vi "Dashboard Main.vi"() -> ()   [LabVIEW 2017]
uses:
  <vilib>/event_ctls.llb/eventvkey.ctl
  <vilib>/Rock Robotics/WPI/Dashboard/WPI_DashboardLogging Global.vi
  <vilib>/Utility/miscctls.llb/LVRowAndColumnTypeDef.ctl
  Shared/TypeDef/Cluster_Drive_RPM.ctl
  Support/Utility/FP_Size VI to Decoration Simple.vi/TypeDefs_Utility/ENUM RB_Pos_Quadrant Position.ctl
  Support/Utility/FP_Size VI to Decoration Simple.vi/TypeDefs_Utility/Cluster_FP Set.ctl
  RoboRio code/TypeDef/CLUSTER_Drive_Point Specification.ctl
panel:
  in  "Camera Settings Right":T1={"Frame Rate"=30, "Compression"=30, "Size"=1, "DB Camera Config"=FALSE} {"Frame Rate" scale=1.0..30.0; "Compression" scale=100.0..-1.0; "Size" items=["640x480", "320x240", "160x120"]}
  in  "Camera Name Right":string(combo)="No Camera Selection"
  out "Camera Info":cluster{"Mbps LED":bool, "Mbps":dbl, "fps":dbl} {"fps" format="%#.1g"; "Mbps" format="%#.1g"}
  in  "Camera Settings":T1={"Frame Rate"=30, "Compression"=30, "Size"=1, "DB Camera Config"=FALSE} {"Frame Rate" scale=1.0..30.0; "Compression" scale=100.0..-1.0; "Size" items=["640x480", "320x240", "160x120"]}
  in  "TCP":refnum<k5>
  in  "Rec Mode":enum32{"Stop", "Record", "Playback"}(radio)
  out "Robot IP":string
  out "Image Message":string="Timeout in Camera Communications"
  in  "Dashboard Tab":T2(tab)
  in  "Select Auto":string(combo)="Select Autonomous ..."
  out "NT Connection":bool
  out "MotorChart R":cluster{"Numeric":dbl, "Numeric":dbl}(graph)
  out "MotorChart L":cluster{"Numeric":dbl, "Numeric":dbl}(graph)
  out "MotorSliders R":cluster{"MotorSlide1":dbl, "MotorSlide2":dbl} {"MotorSlide2" scale=-1.0..1.0 scale format="%#_2e"; "MotorSlide1" scale=-1.0..1.0 scale format="%#_2e"}
  out "MotorSliders L":cluster{"MotorSlide1":dbl, "MotorSlide2":dbl} {"MotorSlide2" scale=-1.0..1.0 scale format="%#_2e"; "MotorSlide1" scale=-1.0..1.0 scale format="%#_2e"}
  out "Gyro":dbl(knob) scale=0.0..360.0
  out "JS1 Z":dbl(slide) scale=-1.0..1.0 scale format="%#_2e"
  out "JS1 Graph":cluster{"X":dbl, "Y":dbl}[](graph)
  out "JS1 Buttons":T3
  out "JS2 Z":dbl(slide) scale=-1.0..1.0 scale format="%#_2e"
  out "JS2 Graph":cluster{"X":dbl, "Y":dbl}[](graph)
  out "JS2 Buttons":T3
  out "Mode":T4(ring)=enum."Auto Disabled"
  out "Camera Image Right":T5(plugin-control)
  in  "DB/String 9":string
  in  "DB/String 8":string
  in  "DB/String 7":string
  in  "DB/String 6":string
  in  "DB/String 5":string
  in  "DB/String 4":string
  in  "DB/String 3":string
  in  "DB/String 2":string
  in  "DB/String 1":string
  in  "DB/String 0":string
  in  "DB/Slider 0":dbl(slide) scale=0.0..5.0
  in  "DB/Slider 1":dbl(slide) scale=0.0..5.0
  in  "DB/Slider 2":dbl(slide) scale=0.0..5.0
  in  "DB/Slider 3":dbl(slide) scale=0.0..5.0
  out "DB/LED 3":bool
  out "DB/LED 2":bool
  out "DB/LED 1":bool
  out "DB/LED 0":bool
  in  "DB/Button 3":bool
  in  "DB/Button 2":bool
  in  "DB/Button 1":bool
  in  "DB/Button 0":bool caption="New Name"
  out "Low Gear":bool
  out "High Gear":bool
  out "Drive Mode":enum16{"Motion Profile", "VBus", "Stop"}(ring)
  out "Profile Enabled":bool
  out "Turbo Enabled":bool
  out "VBus X":dbl
  out "VBus Y":dbl
  out "Right Encoder":dbl
  out "Left Encoder":dbl
  out "Comp. Running":bool
  out "Comp. Enabled":bool
  in  "Reset Max RPM":bool
  out "Right Max":dbl
  out "Left Max":dbl
  out "Right":dbl
  out "Left":dbl
  out "Left Front":dbl
  out "Right Back":dbl
  out "Right Front":dbl
  out "Left Back":dbl
  out "Battery Meter":dbl(knob) scale=0.0..15.0
  out "Solenoid":bool[](array[boolean])
  out "Batt V":bool
  out "Temp":bool
  out "HW":bool
  out "Comp.":bool
  out "Voltage(V)":dbl
  out "Power (W)":dbl
  out "Energy (J)":dbl
  out "Input (V)":dbl
  out "Solenoid (V)":dbl
  out "Current (A)":dbl
  out "5V Usr. Rail Brn.":bool
  out "Input Brn.":bool
  out "6V":bool
  out "3.3V":bool
  out "5V":bool
  out "?":T6(graph)
  out "?":T6(graph)
  out "PDP Currents":string[][](table)
  in  "Profule Array":T7[](array[typedef])
  in  "Send Profile to RIO":bool
  out "Import Successful":bool
  in  "Prifile File Path on PC":path
  in  "Import File":bool
  in  "Test Slider":dbl(slide) scale=0.0..100.0 scale format="%#_3g"
  in  "On/Off":bool caption="Solenoid"
  in  "Test Name":u16(ring) items=["Select the test to run..."]
  in  "Test Tree":string(tree)
  in  "Motor":cluster{"Value":dbl, "Enable":bool} {"Value" scale=-1.0..1.0 scale format="%#_3g"}
  out "Progress":T8 {"Test Progress" scale=0.0..100.0}
  in  "Rev/Fwd":cluster{"Forward":bool, "Reverse":bool}
  in  "Test Ring":u16(ring) items=["Monochrome", "Color"]
  out "Cmd Status":string
  in  "Execute Command":bool
  in  "Command Params":string[][](table)
  in  "Command Selection":i32(listbox)
  in  "CheckList":i32(listbox)
  out "Tree":string(tree)
  out "Camera Image":T5(plugin-control)
  in  "Camera Name":string(combo)="No Camera Selection"
  # "HW"
  # "HW"
  # "Joysticks"
  # "Drive Motors"
  # "Front"
  # "Right"
  # "Left"
  # "Back"
  # "SRX Currents"
  # "Drive RPMs"
  # "Drive"
  # "Faults"
  # "PDP"
  # "PCM"
  # "RIO Faults"
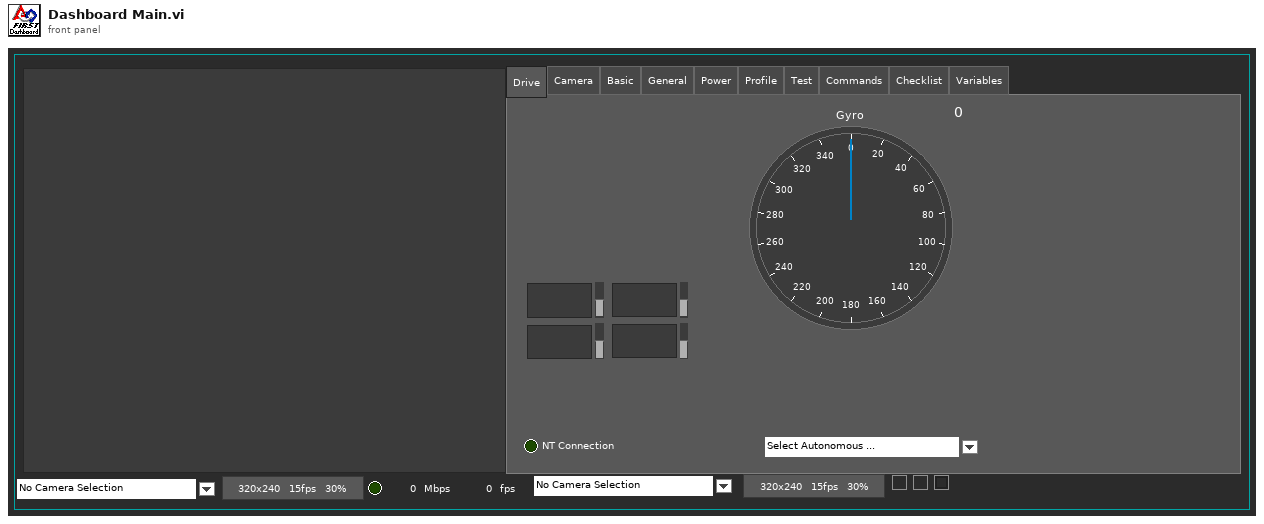
[diagram p1: front panel]
types:
  T1 = cluster{"Frame Rate":i32, "Compression":i32, "Size":u16, "DB Camera Config":bool}
  T2 = enum32{"Drive", "Camera", "Basic", "General", "Power", "Profile", "Test", "Commands", "Checklist", "Variables"}
  T3 = cluster{bool, bool, bool, bool, bool, bool, bool, bool, bool, bool, bool, bool}
  T4 = enum8{"Tele-Op Disabled", "Tele-Op Enabled", "Auto Disabled", "Auto Enabled", "Test Disabled", "Test Enabled", "Disconnected", "No Code", "E-Stop"}
  T5 = typedef "IMAQ Image.ctl" = refnum<image>
  T6 = cluster{"Vol.  (V)":dbl, "Vol.  (V)":dbl, "Vol.  (V)":dbl}
  T7 = typedef "CLUSTER_Drive_Point Specification.ctl" = cluster{"Position":dbl, "Velocity":dbl, "Duration ms":u8}
  T8 = cluster{"Test Progress":u8, "Test Progress Text":string}
  T9 = cluster{"Operation":enum16{"Update", "Clear"}, "Color Box":u32}[]
  T10 = typedef "Image Type" = u32
  T11 = cluster{"IDs":cluster{"RPC field ID":u16, "Unique ID":u16}, "String":string}
  T12 = enum32{"Drive", "Basic", "Custom", "Test", "Checklist", "Variables"}
  T13 = cluster{"Camera Image":refnum<vi>, "Dashboard Tab":refnum<vi>, "Rec Mode":refnum<vi>, "Test Slider":refnum<vi>, "On/Off ":refnum<vi>, "Test Ring":refnum<vi>, "Rev/Fwd":refnum<vi>, "Test Name":refnum<vi>, "Motor":refnum<vi>, "Progress":refnum<vi>, "CheckList":refnum<vi>, "Tree":refnum<vi>, "Test Tree":refnum<vi>, "Command Params":refnum<vi>, "Command Selection":refnum<vi>, "Execute Command":refnum<vi>, "Cmd Status":refnum<vi>, "Camera Settings":refnum<vi>, "Camera Name":refnum<vi>, "Camera Info":refnum<vi>, "Camera Settings Right":refnum<vi>, "Camera Name Right":refnum<vi>, "Camera Image Right":refnum<vi>}
  T14 = typedef "Cluster_FP Set.ctl" = cluster{"Menu Bar":bool, "Position":T15, "Decoration index":i32, "border(px)":i32, "Monitor #":i32}
  T15 = typedef "ENUM RB_Pos_Quadrant Position.ctl" = enum32{"LFT-TOP", "MID-TOP", "RGT-TOP", "LFT-CTR", "MID-CTR", "RGT-CTR", "LFT-BOT", "MID-BOT", "RGT-BOT"}
  T16 = typedef "Cluster_Drive_RPM.ctl" = cluster{"Left Side":dbl, "Right Side":dbl}
  T17 = typedef "LVRowAndColumnTypeDef.ctl" = cluster{"Row":i32, "Column":i32}
  T18 = cluster{"Error Strings":string, "Disable Counts":cluster{u16, u16}, "Rail Faults":cluster{u16, u16, u16}, "Robot IP":string, "DB Mode":u8, "Event Info":cluster{"Name":string, "Type":u8, "Number":u16, "Replay":u8}}
  T19 = cluster{"Storage":cluster{"Disk Free":u64, "RAM Block":u32, "RAM free":u32}, "CPU Utilization":cluster{"CPU % ISR":sgl, "CPU % Time Crit":sgl, "CPU % Timed Str":sgl, "CPU % High":sgl, "CPU % Above":sgl, "CPU % Normal":sgl, "CPU % Low":sgl}, "CAN":cluster{"% Bus Utilization":sgl, "Bus Off Cnt":u32, "TX_FIFO Full Cnt":u32, "Receive Error Cnt":u8, "Transmit Error Cnt":u8}, "HID":cluster{"HID Outputs":u32, "Rumble Low":u16, "Rumble High":u16}[]}
  T20 = cluster{"Status bits":cluster{"Test Mode":bool, "Autonomous":bool, "Enabled":bool, "Code Start":bool, "Brownout":bool, "Reserved 2":bool, "Reserved 3":bool, "E-Stop":bool}, "Code Trace":cluster{"Disabled":bool, "TeleOp":bool, "Auto":bool, "Test":bool}, "Controller Type":enum16{"unknown", "cRIO", "roboRio"}, "Code?":enum16{"unknown", "noCode", "code"}, "Battery V":dbl}
  T21 = cluster{"Control Bits":cluster{"TestMode":bool, "Autonomous":bool, "Enabled":bool, "FMS Present":bool, bool, bool, bool, "E-Stop":bool}, "Team Station ":u8, "Countdown":sgl, "Joystick Values":cluster{"Axes":dbl[], "Buttons":bool[], "POVs":i16[]}[]}
  T22 = cluster{"Axes":dbl[], "Buttons":bool[], "POVs":i16[]}[]
  T23 = typedef "CLUSTER_PDP_Status.ctl" = cluster{"PDP Faults":T24, "All Currents (A)":dbl[], "Energy (J)":dbl, "Power (W)":dbl, "Voltage (V)":dbl}
  T24 = typedef "CLUSTER_PDP_Faults.ctl" = cluster{"Current Faults":bool[], "Batt V Fault":bool, "Temp Fault":bool, "HW Fault":bool}
  T25 = typedef "CLUSTER_PCM_Status.ctl" = cluster{"Current (A)":dbl, "All Solenoid Faults":bool[], "Input Voltage":dbl, "Solenoid Voltage":dbl, "Comp. Fault":bool}
  T26 = typedef "CLUSTER_RoboRio_Status.ctl" = cluster{"RoboRio Faults":T27, "RIO inpt vol (V)":dbl, "RIO inpt cur (A)":dbl, "RoboRio Rails":T28}
  T27 = typedef "CLUSTER_RoboRio_Faults.ctl" = cluster{"Inpt. V. Brn. Out":bool, "3.3V Usr Rail Shrt.":bool, "5 V Usr Rail Shrt.":bool, "6 V Usr. Rail Shrt.":bool, "5V Usr. Rail Brn. Out":bool}
  T28 = typedef "CLUSTER_RoboRio_Rails.ctl" = cluster{"3.3 Volt":T29, "5 Volt":T29, "6 Volt":T29}
  T29 = typedef "CLUSTER_RoboRio_SingleRail.ctl" = cluster{"Vol.  (V)":dbl, "Cur. (A)":dbl}
  T30 = cluster{"Axes":dbl[], "Buttons":bool[], "POVs":i16[]}
  T31 = cluster{"Buttons[0]":bool, "Buttons[1]":bool, "Buttons[2]":bool, "Buttons[3]":bool, "Buttons[4]":bool, "Buttons[5]":bool, "Buttons[6]":bool, "Buttons[7]":bool, "Buttons[8]":bool, "Buttons[9]":bool, "Buttons[10]":bool, "Buttons[11]":bool}
  T32 = cluster{"Cur. (A)":dbl, "Cur. (A)":dbl, "Cur. (A)":dbl}
  T33 = typedef "Cluster_SRX_Amperage.ctl" = cluster{"Left Back":dbl, "Right Front":dbl, "Right Back":dbl, "Left Front":dbl}
  T34 = typedef "Cluster_Compressor.ctl" = cluster{"Compressor Running":bool, "Compressor Enabled":bool}
  T35 = typedef "Cluster_Encoder_Count.ctl" = cluster{"Left Side Encoder":dbl, "Right Side Encoder":dbl}
  T36 = typedef "CLUSTER_CMD_WC_Drive.ctl" = cluster{"Drive_Mode":T37, "VBus":T38, "Profile":T40}
  T37 = typedef "ENUM_WC_Drive_DriveMode.ctl" = enum16{"Motion Profile", "VBus", "Stop"}
  T38 = typedef "CLUSTER_Drive_ACT Loop_VBus Data.ctl" = cluster{"Drive":T39, "Turbo":bool}
  T39 = typedef "CLUSTER_X and Y.ctl" = cluster{"Steer":dbl, "Throtle":dbl}
  T40 = typedef "CLUSTER_Drive_ACT Loop_Profile Data.ctl" = cluster{"Start":bool}
  T41 = cluster{"Command Params":string[][], "Test Mode Array":cluster{"Operation":enum16{"Update", "Clear"}, "Color Box":u32}[]}
  T42 = typedef "eventvkey.ctl" = enum16{"ASCII", "Enter", "Return", "Shift", "Ctrl", "Alt", "Cmd", "Opt", "Caps", "NumLock", "Clear", "Break", "Up", "Down", "Left", "Right", "Insert", "Delete", "Home", "End", "PageUp", "PageDown", "Escape", "Help", "Pause", "ScrollLock", "F1", "F2", "F3", "F4", "F5", "F6", "F7", "F8", "F9", "F10", "F11", "F12", "F13", "F14", "F15", "F16", "F17", "F18", "F19", "F20", "F21", "F22", "F23", "F24", "Play", "VolumeUp", "VolumeDown", "Mute", "Two Byte Char"}
  T43 = cluster{"Image Size":bool, "Image Type":bool, "Pixel Value":bool, "ROI Information":bool, "Zoom Factor":bool}
  T44 = cluster{"Operation":enum16{"Update", "Clear"}, "Color Box":u32}
  T45 = cluster{"Shift":bool, "Ctrl":bool, "Alt":bool, "Cmd":bool, "Opt":bool}
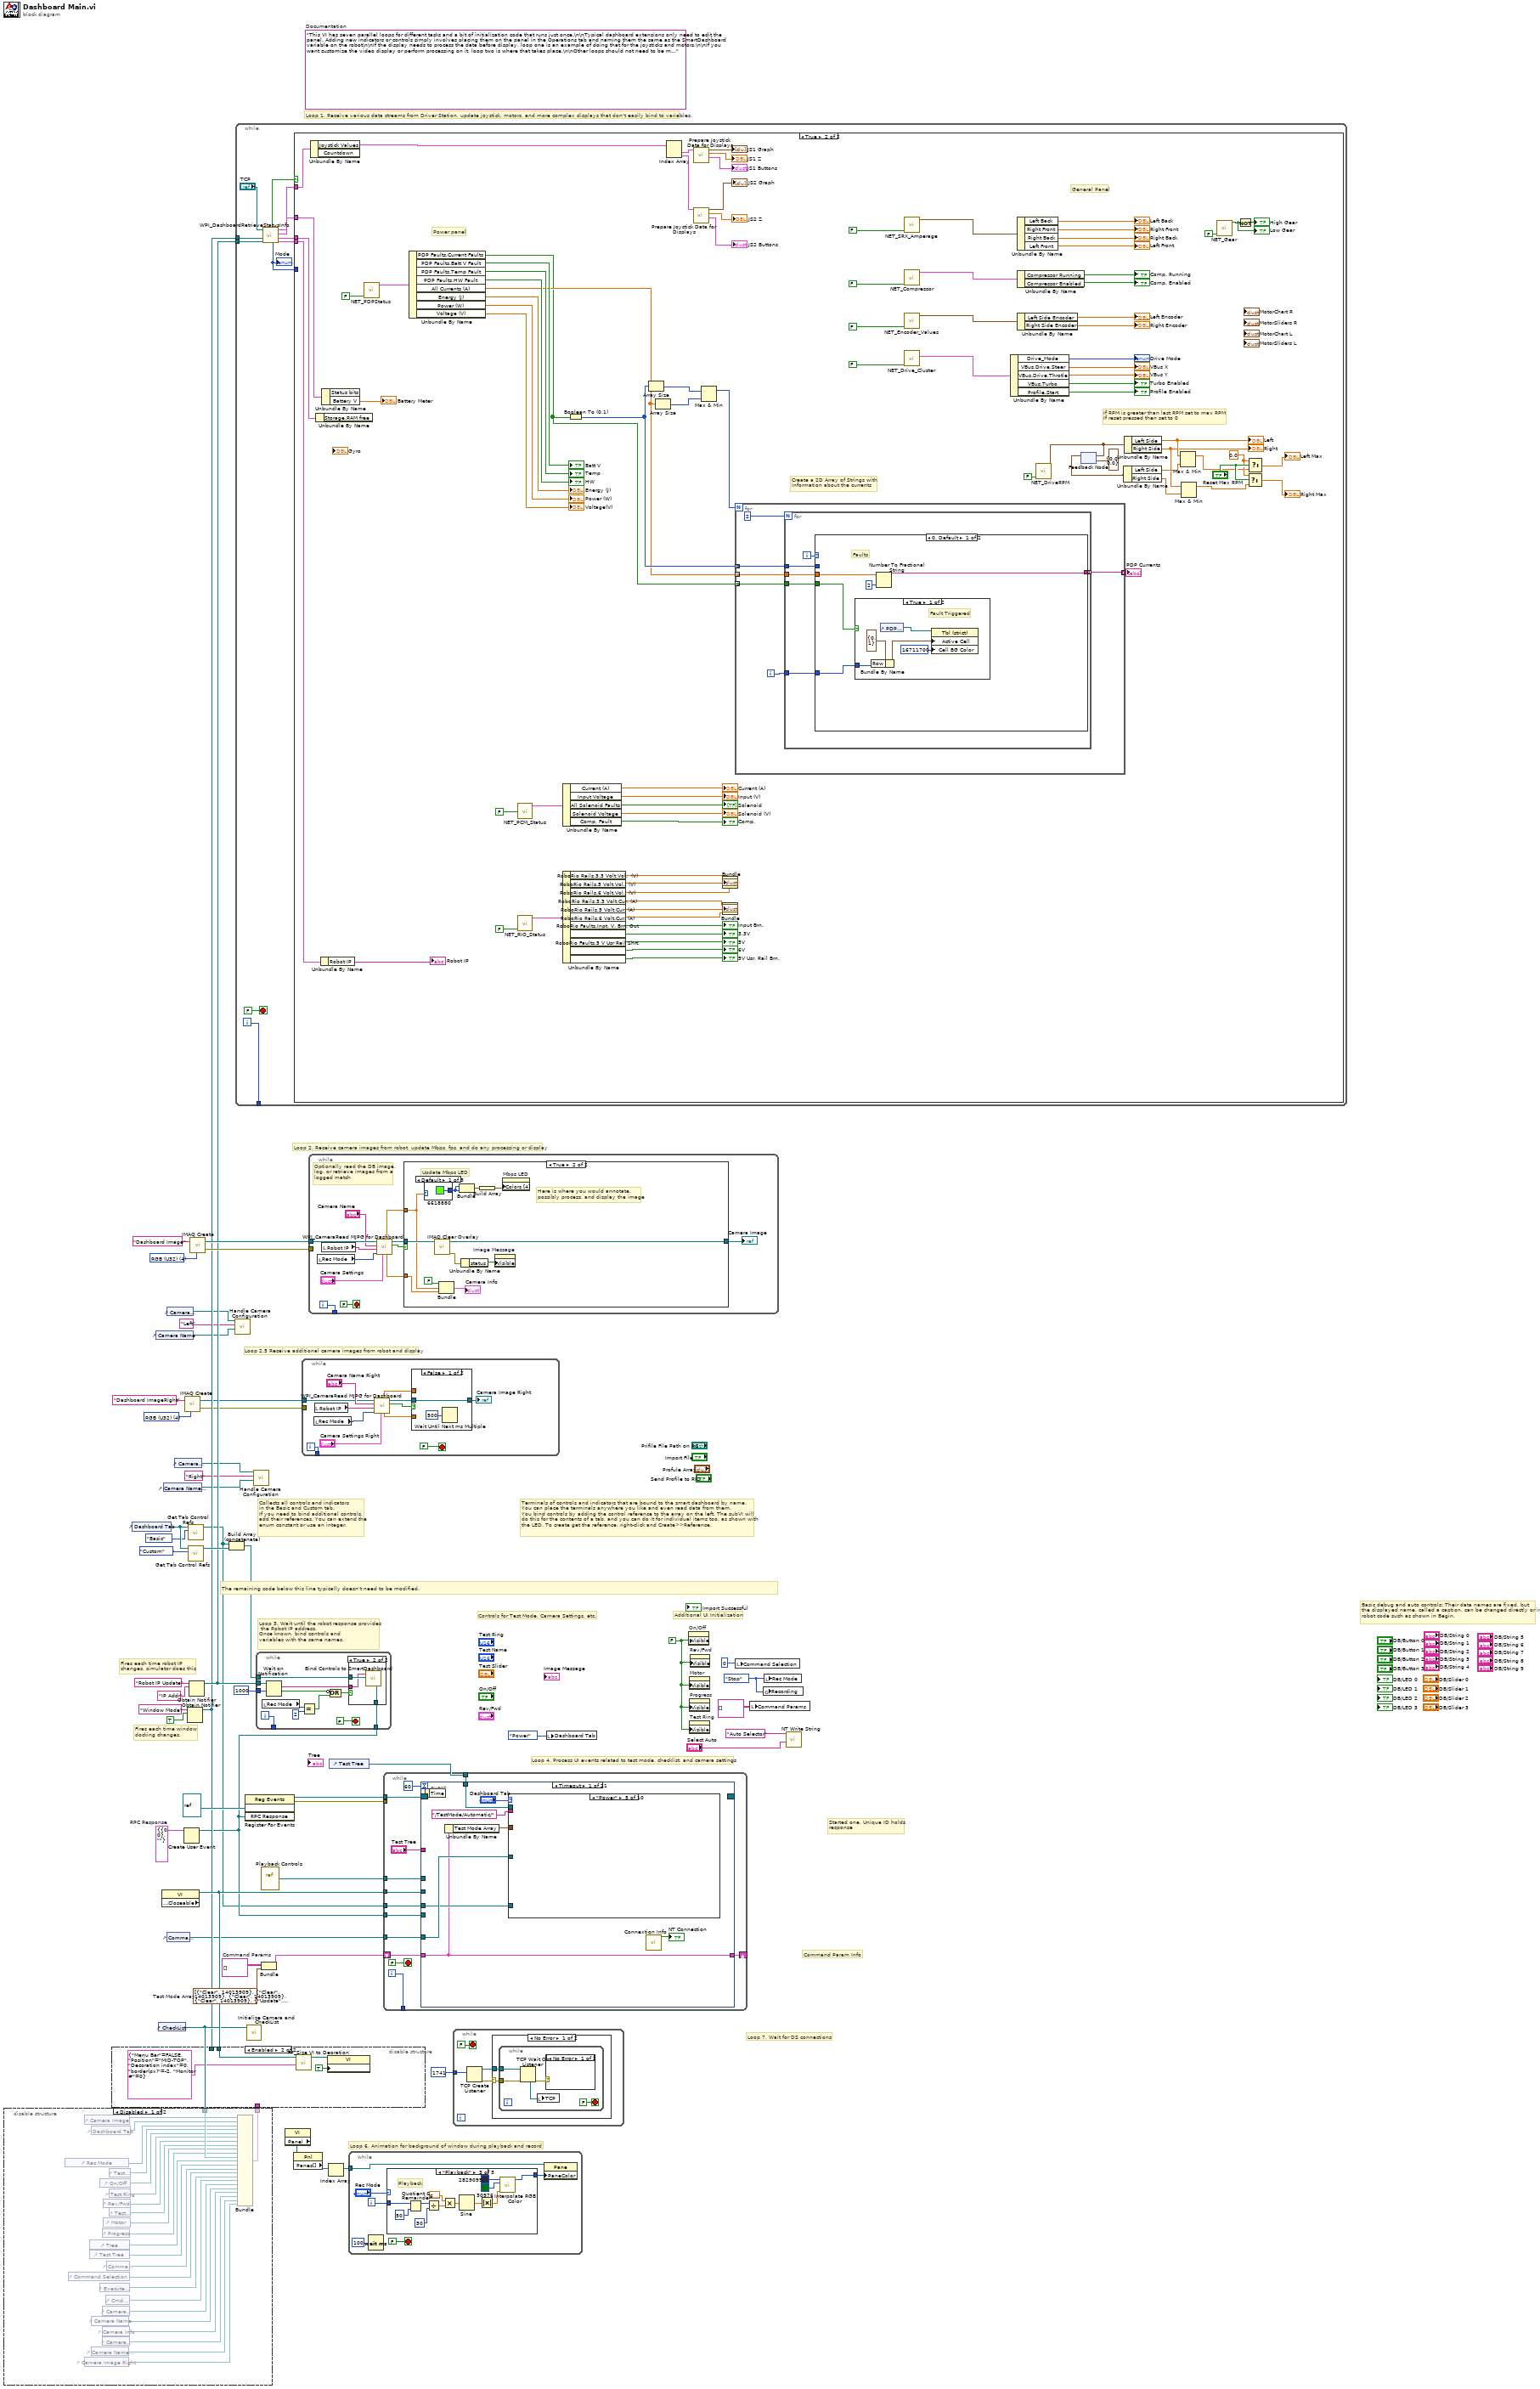
[diagram p0: block diagram]
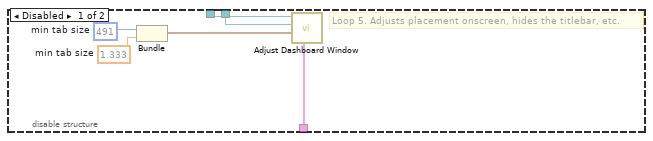
[diagram p2: hidden frame]
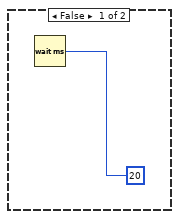
[diagram p5: hidden frame]
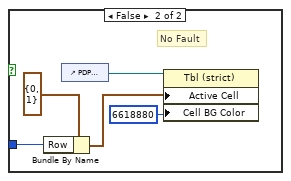
[diagram p6: hidden frame]
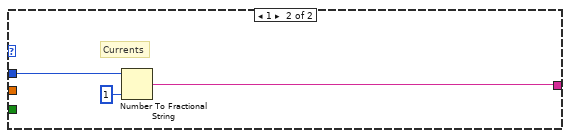
[diagram p7: hidden frame]
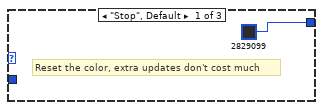
[diagram p8: hidden frame]
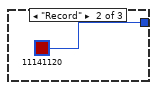
[diagram p9: hidden frame]
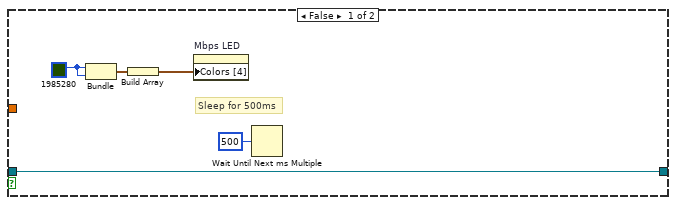
[diagram p11: hidden frame]
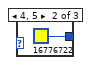
[diagram p12: hidden frame]
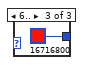
[diagram p13: hidden frame]
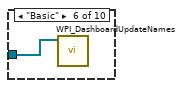
[diagram p18: hidden frame]
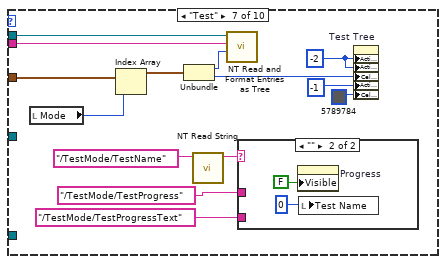
[diagram p19: hidden frame]
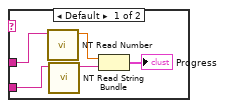
[diagram p20: hidden frame]
diagram:
  w2 = T9 [{"Operation"=enum."Clear", "Color Box"=14013909}, {"Operation"=enum."Clear", "Color Box"=14013909}, {"Operation"=enum."Clear", "Color Box"=14013909}, {"Operation"=enum."Clear", "Color Box"=14013909}, {"Operation"=enum."Update", "Color Box"=14013909}, {"Operation"=enum."Update", "Color Box"=16777215}, {"Operation"=enum."Clear", "Color Box"=14013909}, {"Operation"=enum."Clear", "Color Box"=14013909}, {"Operation"=enum."Clear", "Color Box"=14013909}]  # Test Mode Array
  w4 = string[][] []  # Command Params
  w11 = T10 4 items=["Grayscale (U8)", "Grayscale (I16)", "Grayscale (SGL)", "Complex (CSG)", "RGB (U32)", "HSL (U32)", "RGB (U64)"] ("Image Type")
  w22 = T11 {"IDs"={"RPC field ID"=0, "Unique ID"=0}, "String"=""}  # RPC Response
  w35 = enum32{"Stop", "Record", "Playback"}."Stop" ("Rec Mode")
  w26 = FALSE ("Visible")
  (unwired) "This VI has seven parallel loops for different tasks and a bit of initialization code that runs just once.\n\nTypical dashboard extensions only need to edit the panel. Adding new indicators or controls simply involves placing them on the panel in the Operations tab and naming them the same as the SmartDashboard variable on the robot\n\nIf the display needs to process the data before display, loop one is an example of doing that for the joysticks and motors.\n\nIf you want customize the video display or perform processing on it, loop two is where that takes place.\n\nOther loops should not need to be modified. They are pretty standard, and document the task they perform."  # Documentation
  w52 = T10 4 items=["Grayscale (U8)", "Grayscale (I16)", "Grayscale (SGL)", "Complex (CSG)", "RGB (U32)", "HSL (U32)", "RGB (U64)"] ("Image Type")
  # "Loop 2.5 Receive additional camera images from robot and display"
  # "Command Param Info"
  # "Started one, Unique ID holds\nresponse"
  # "Loop 7. Wait for DS connections"
  # "Basic debug and auto controls: Their data names are fixed, but\nthe displayed name, called a caption, can be changed directly or in\nrobot code such as shown in Begin."
  # "Controls for Test Mode, Camera Settings, etc."
  # "Additional UI Initialization"
  # "Loop 6. Animation for background of window during playback and record"
  # "Fires each time robot IP\nchanges, simulator does this"
  # "Fires each time window\ndocking changes."
  # "Collects all controls and indicators\nin the Basic and Custom tab.\nIf you need to bind additional controls,\nadd their references. You can extend the\nenum constant or use an integer."
  # "The remaining code below this line typically doesn't need to be modified."
  # "Loop 4. Process UI events related to test mode, checklist, and camera settings"
  # "Terminals of controls and indicators that are bound to the smart dashboard by name.\nYou can place the terminals anywhere you like and even read data from them.\nYou bind controls by adding the control reference to the array on the left. The subVI will\ndo this for the contents of a tab, and you can do it for individual items too, as shown with\nthe LED. To create get the reference, right-click and Create>>Reference."
  # "Loop 3. Wait until the robot response provides\n the Robot IP address.\nOnce known, bind controls and\nvariables with the same names."
  # "Loop 1. Receive various data streams from Driver Station, update joystick, motors, and more complex displays that don't easily bind to variables."
  # "Loop 2. Receive camera images from robot, update Mbps, fps, and do any processing or display"
  n1 = control-ref of="Dashboard Tab"() -> (w33:refnum<vi>)
  n2 = control-ref of="Camera Name"() -> (w16:refnum<vi>)
  n3 = control-ref of="CheckList"() -> (w27:refnum<vi>)
  n4 = disable-structure shown="Disabled" {
    disable-tunnel: [w74 _] -> w28
    disable-tunnel: w27 -> [w73 _]
    frame Disabled {
      n5 = control-ref of="Rec Mode"() -> (w68:refnum<vi>)
      n6 = control-ref of="Command Selection"() -> (w60:refnum<vi>)
      n7 = control-ref of="Camera Image Right"() -> (w53:refnum<vi>)
      n8 = control-ref of="Camera Image"() -> (w76:refnum<vi>)
      n9 = control-ref of="Tree"() -> (w72:refnum<vi>)
      n10 = control-ref of="Test Tree"() -> (w71:refnum<vi>)
      n11 = control-ref of="Dashboard Tab"() -> (w75:refnum<vi>)
      n12 = control-ref of="Camera Name"() -> (w57:refnum<vi>)
      n13 = control-ref of="Camera Name Right"() -> (w54:refnum<vi>)
      n14 = control-ref of="Execute Command"() -> (w61:refnum<vi>)
      n15 = control-ref of="On/Off"() -> (w66:refnum<vi>)
      n16 = control-ref of="Progress"() -> (w63:refnum<vi>)
      n17 = control-ref of="Camera Settings"() -> (w58:refnum<vi>)
      n18 = control-ref of="Camera Info"() -> (w56:refnum<vi>)
      n19 = control-ref of="Camera Settings Right"() -> (w55:refnum<vi>)
      n20 = control-ref of="Rev/Fwd"() -> (w64:refnum<vi>)
      n21 = control-ref of="Motor"() -> (w69:refnum<vi>)
      n22 = control-ref of="Cmd Status"() -> (w59:refnum<vi>)
      n23 = control-ref of="Command Params"() -> (w62:refnum<vi>)
      n24 = control-ref of="Test Slider"() -> (w67:refnum<vi>)
      n25 = control-ref of="Test Ring"() -> (w65:refnum<vi>)
      n26 = control-ref of="Test Name"() -> (w70:refnum<vi>)
      n27 = Bundle("Camera Image"=w76, "Dashboard Tab"=w75, "Rec Mode"=w68, "Test Slider"=w67, "On/Off"=w66, "Test Ring"=w65, "Rev/Fwd"=w64, "Test Name"=w70, "Motor"=w69, "Progress"=w63, "CheckList"=w73, "Tree"=w72, "Test Tree"=w71, "Command Params"=w62, "Command Selection"=w60, "Execute Command"=w61, "Cmd Status"=w59, "Camera Settings"=w58, "Camera Name"=w57, "Camera Info"=w56, "Camera Settings Right"=w55, "Camera Name Right"=w54, "Camera Image Right"=w53) -> (w74:T13)  [unwired: 1 in]
    }
    frame Enabled {
    }
  }
  n28 = property class="VI" props=["Front Panel.Closeable"]() -> (reference out=w34:refnum<vi>)  [unwired: 2 in, 2 out]
  n29 = control-ref of="Camera Name Right"() -> (w7:refnum<vi>)
  n30 = control-ref of="Camera Settings"() -> (w17:refnum<vi>)
  n31 = control-ref of="Command Params"() -> (w18:refnum<vi>)
  n32 = control-ref of="Camera Settings Right"() -> (w8:refnum<vi>)
  n33 = Create User Event(user event datatype=w22) -> (user event=w19:refnum<user-event>)  [unwired: 1 in, 1 out]
  n34 = call "IMAQ Create"("Image Name"="Dashboard ImageRight", "Image Type"=w11) -> ("New Image"=w10:T5, "error out"=w9:errorcluster)  [unwired: 2 in, 1 out]
  n35 = Obtain Notifier(name (unnamed)="Window Mode", notification data type=TRUE) -> (notifier out=w24:refnum<notifier>)  [unwired: 2 in, 2 out]
  n36 = disable-structure shown="Enabled" {
    disable-tunnel: w34 -> [w82 w86]
    disable-tunnel: w28 -> [w78 _]
    disable-tunnel: w24 -> [w77 _]
    frame Disabled {
      w81 = 491  # min tab size
      w80 = 1.333  # min tab size
      # "Loop 5. Adjusts placement onscreen, hides the titlebar, etc."
      n37 = Bundle("min tab size"=w81, "min tab size"=w80) -> (w79:cluster{"min tab size":i32, "min tab size":dbl})  [unwired: 1 in]
      n38 = call "Adjust Dashboard Window.vi"("Sizing Refnums"=w78, "Size Constraints"=w79, "VI"=w82, "WIn Mode"=w77) -> ()  [unwired: 8 in]
    }
    frame Enabled {
      n39 = call "FP_Size VI to Deoration.vi"("FPSet"=T14 {"Menu Bar"=FALSE, "Position"=enum."MID-TOP", "Decoration index"=0, "border(px)"=-2, "Monitor #"=0}, "VI Ref"=w86) -> ("VI Ref Out"=w84:refnum<vi>)  [unwired: 8 in, 1 out]
      n40 = property class="VI"(reference=w84, "Front Panel.IsFrontmost"=TRUE ("Front Panel Window:Is Frontmost")) -> ()  [unwired: 1 in, 2 out]
    }
  }
  n41 = call <vilib>:"Get Tab Control Refs.vi"("Page Index"=T12."Basic" ("Dashboard Tab"), "TabControl in"=w33) -> ("ControlsOnPage"=w15:refnum<vi>[])  [unwired: 9 in]
  n42 = call <vilib>:"Get Tab Control Refs.vi"("Page Index"=T12."Custom" ("Dashboard Tab"), "TabControl in"=w33) -> ("ControlsOnPage"=w32:refnum<vi>[])  [unwired: 9 in]
  n43 = Obtain Notifier(name (unnamed)="Robot IP Update", notification data type="IP Addr" ("name (unnamed)")) -> (notifier out=w25:refnum<notifier>)  [unwired: 2 in, 2 out]
  n44 = call "IMAQ Create"("Image Name"="Dashboard Image", "Image Type"=w52) -> ("New Image"=w50:T5, "error out"=w49:errorcluster)  [unwired: 2 in, 1 out]
  n45 = Build Array (concatenate)(w15, w32) -> (w31:refnum<vi>[])
  n46 = call "Handle Camera Configuration.vi"("CameraNameRef"=w16, "Camera File Name"="Left", "ClusterRef"=w17) -> ()  [unwired: 9 in]
  n47 = while {
    tunnel: [w96] -> _
    tunnel: w25 -> [w90]
    tunnel: w24 -> [w87]
    i -> [w96]
    stop <- FALSE stop-if-true
    n48 = call <vilib>:"WPI_DashboardRetrieveStatusInfo.vi"("Binding Refnum"=w90, "Window Mode Notifier"=w87, "TCP Cnx"="TCP") -> ("Power and Errors"=w91:T18, "Robot Metrics"=w94:T19, "Status Info"=w95:T20, "Control Info"=w92:T21, "Robot Mode"=w89:T4, "Process?"=w93:bool)  [unwired: 3 in]
    "Mode" <- w89
    n49 = case shown="True" w93 {
      tunnel: w95 -> [_ w188]
      tunnel: w94 -> [_ w187]
      tunnel: w92 -> [_ w186]
      tunnel: w91 -> [_ w185]
      tunnel: w89 -> [_ _]
      frame False {
        n50 = Wait (ms)(milliseconds to wait=u32 20) -> ()  [unwired: 1 out]
      }
      frame True {
        w108 = 0.0 ("t")
        # "Power panel"
        # "Create a 2D Array of Strings with \ninformation about the currents"
        # "General Panel"
        # "If RPM is greater than last RPM set to max RPM\nIf reset pressed then set to 0"
        n51 = Unbundle By Name(w186) -> ("Joystick Values"=w184:T22)  [unwired: 1 out]
        n52 = Unbundle By Name(w187) -> ()  [unwired: 1 out]
        n53 = Unbundle By Name(w185) -> ("Robot IP"=→"Robot IP":string)
        n54 = Unbundle By Name(w188) -> ("Battery V"=→"Battery Meter":dbl)  [unwired: 1 out]
        n55 = call "NET_PDPStatus.vi"("Read(F) Write(T)"=FALSE) -> ("PDP_Status_Out"=w146:T23)  [unwired: 10 in]
        n56 = Unbundle By Name(w146) -> ("PDP Faults.Current Faults"=w115:bool[], "PDP Faults.Batt V Fault"=→"Batt V":bool, "PDP Faults.Temp Fault"=→"Temp":bool, "PDP Faults.HW Fault"=→"HW":bool, "All Currents (A)"=w137:dbl[], "Energy (J)"=→"Energy (J)":dbl, "Power (W)"=→"Power (W)":dbl, "Voltage (V)"=→"Voltage(V)":dbl)
        n57 = call "NET_PCM_Status.vi"("Read(F) Write(T)"=FALSE) -> ("PCM_Status_Out"=w152:T25)  [unwired: 10 in]
        n58 = call "NET_RIO_Status.vi"("Read(F) Write(T)"=FALSE) -> ("RoboRio Status Out"=w162:T26)  [unwired: 10 in]
        n59 = Unbundle By Name(w152) -> ("Current (A)"=→"Current (A)":dbl, "Input Voltage"=→"Input (V)":dbl, "All Solenoid Faults"=→"Solenoid":bool[], "Solenoid Voltage"=→"Solenoid (V)":dbl, "Comp. Fault"=→"Comp.":bool)
        n60 = Unbundle By Name(w162) -> ("RoboRio Rails.3.3 Volt.Vol.  (V)"=w166:dbl, "RoboRio Rails.5 Volt.Vol.  (V)"=w165:dbl, "RoboRio Rails.6 Volt.Vol.  (V)"=w164:dbl, "RoboRio Rails.3.3 Volt.Cur. (A)"=w160:dbl, "RoboRio Rails.5 Volt.Cur. (A)"=w161:dbl, "RoboRio Rails.6 Volt.Cur. (A)"=w159:dbl, "RoboRio Faults.Inpt. V. Brn. Out"=→"Input Brn.":bool, "RoboRio Faults.3.3V Usr Rail Shrt."=→"3.3V":bool, "RoboRio Faults.5 V Usr Rail Shrt."=→"5V":bool, "RoboRio Faults.6 V Usr. Rail Shrt."=→"6V":bool, "RoboRio Faults.5V Usr. Rail Brn. Out"=→"5V Usr. Rail Brn.":bool)
        n61 = Boolean To (0,1)(Boolean=w115) -> (0, 1=w138:i16[])
        n62 = Array Size(array=w138) -> (size(s)=w139:i32)
        n63 = Array Size(array=w137) -> (size(s)=w118:i32)
        n64 = Index Array(array=w184) -> (element #1=w183:T30, element #2=w179:T30)  [unwired: 2 in]
        n65 = call "Prepare Joystick Data for Displays.vi"("Joystick Values"=w179) -> ("Buttons"=→"JS2 Buttons":T31, "Z Axis"=→"JS2 Z":dbl, "Cartesian Data"=→"JS2 Graph":cluster{"X axis":dbl, "X axis":dbl}[])  [unwired: 8 in]
        n66 = call "Prepare Joystick Data for Displays.vi"("Joystick Values"=w183) -> ("Buttons"=→"JS1 Buttons":T31, "Z Axis"=→"JS1 Z":dbl, "Cartesian Data"=→"JS1 Graph":cluster{"X axis":dbl, "X axis":dbl}[])  [unwired: 8 in]
        n67 = Max & Min(x=w139, y=w118) -> (max(x,y)=w117:i32)  [unwired: 1 out]
        n68 = Bundle("Vol.  (V)"=w166, "Vol.  (V)"=w165, "Vol.  (V)"=w164) -> (→"?":T6)  [unwired: 1 in]
        n69 = Bundle("Cur. (A)"=w160, "Cur. (A)"=w161, "Cur. (A)"=w159) -> (→"?":T32)  [unwired: 1 in]
        n70 = for {
          N: w117 -> [_]
          tunnel: w138 -> [w194] mode=indexing
          tunnel: w137 -> [w192] mode=indexing
          tunnel: [w193] -> w136 mode=indexing
          tunnel: w115 -> [w190] mode=indexing
          i -> [w189]
          n71 = for {
            N: 2 -> [_]
            tunnel: [w199] -> w193 mode=indexing
            tunnel: w194 -> [w200]
            tunnel: w192 -> [w197]
            tunnel: w190 -> [w196]
            tunnel: w189 -> [w195]
            i -> [w198]
            n72 = case shown="0, Default" w198 {
              tunnel: w200 -> [_ w218]
              tunnel: [w204 w217] -> w199
              tunnel: w197 -> [w205 _]
              tunnel: w196 -> [w201 _]
              tunnel: w195 -> [w202 _]
              frame 0, Default {
                # "Faults"
                n73 = case shown="True" w201 {
                  tunnel: w202 -> [w209 w211]
                  frame True {
                    # "Fault Triggered"
                    n74 = Bundle By Name(cluster=T17 {"Row"=0, "Column"=1} ("Active Cell:Active Cell"), "Row"=w209) -> (w207:T17)
                    n75 = control-ref of="PDP Currents"() -> (w206:refnum<vi>)
                    n76 = property class="Tbl (strict)"(reference=w206, "Active Cell"=w207, "Cell BG Color"=u32 16711700 ("Active Cell:Cell Background Color")) -> ()  [unwired: 1 in, 2 out]
                  }
                  frame False {
                    # "No Fault"
                    n77 = Bundle By Name(cluster=T17 {"Row"=0, "Column"=1} ("Active Cell:Active Cell"), "Row"=w211) -> (w213:T17)
                    n78 = control-ref of="PDP Currents"() -> (w212:refnum<vi>)
                    n79 = property class="Tbl (strict)"(reference=w212, "Active Cell"=w213, "Cell BG Color"=u32 6618880 ("Active Cell:Cell Background Color")) -> ()  [unwired: 1 in, 2 out]
                  }
                }
                n80 = Number To Fractional String(number=w205, precision (6)=i16 2) -> (F-format string=w204:string)  [unwired: 2 in]
              }
              frame 1 {
                # "Currents"
                n81 = Number To Fractional String(number=w218, precision (6)=i16 1) -> (F-format string=w217:string)  [unwired: 2 in]
              }
            }
          }
        }
        "PDP Currents" <- w136
        n82 = call "NET_SRX_Amperage.vi"("Read(F) Write(T)"=FALSE) -> ("SRX_Amp_Cluster Out"=w134:T33)  [unwired: 10 in]
        n83 = call "NET_Compressor.vi"("Read(F) Write(T)"=FALSE) -> ("Compressor Out"=w114:T34)  [unwired: 10 in]
        n84 = call "NET_Encoder_Values.vi"("Read(F) Write(T)"=FALSE) -> ("Encoder Counts Out"=w127:T35)  [unwired: 10 in]
        n85 = call "NET_Drive_Cluster.vi"("Read(F) Write(T)"=FALSE) -> ("CMD_DriveCluster Out"=w124:T36)  [unwired: 10 in]
        n86 = Unbundle By Name(w124) -> ("Drive_Mode"=→"Drive Mode":T37, "VBus.Drive.Steer"=→"VBus X":dbl, "VBus.Drive.Throtle"=→"VBus Y":dbl, "VBus.Turbo"=→"Turbo Enabled":bool, "Profile.Start"=→"Profile Enabled":bool)
        n87 = Unbundle By Name(w134) -> ("Left Back"=→"Left Back":dbl, "Right Front"=→"Right Front":dbl, "Right Back"=→"Right Back":dbl, "Left Front"=→"Left Front":dbl)
        n88 = Unbundle By Name(w114) -> ("Compressor Running"=→"Comp. Running":bool, "Compressor Enabled"=→"Comp. Enabled":bool)
        n89 = Unbundle By Name(w127) -> ("Left Side Encoder"=→"Left Encoder":dbl, "Right Side Encoder"=→"Right Encoder":dbl)
        n90 = call "NET_DriveRPM.vi"("Read(F) Write(T)"=FALSE) -> ("Drive RPM Out"=w113:T16)  [unwired: 10 in]
        n91 = feedback-in #1(w113) -> ()
        n92 = feedback #1(T16 {"Left Side"=0.0, "Right Side"=0.0} ("Drive RPM Out")) -> (w112:T16)
        n93 = Unbundle By Name(w112) -> ("Left Side"=w103:dbl, "Right Side"=w99:dbl)
        n94 = Unbundle By Name(w113) -> ("Left Side"=w104:dbl, "Right Side"=w100:dbl)
        "Left" <- w104
        "Right" <- w100
        n95 = Max & Min(x=w104, y=w103) -> (max(x,y)=w102:dbl)  [unwired: 1 out]
        n96 = Max & Min(x=w100, y=w99) -> (max(x,y)=w101:dbl)  [unwired: 1 out]
        n97 = call "NET_Gear.vi"("Read(F) Write(T)"=FALSE) -> ("High Gear Out"=w105:bool)  [unwired: 10 in]
        "Low Gear" <- w105
        n98 = Not(x=w105) -> (.not. x?=→"High Gear":bool)
        n99 = Select(t=w108, s="Reset Max RPM", f=w101) -> (s? t:f=→"Right Max":dbl)
        n100 = Select(t=w108, s="Reset Max RPM", f=w102) -> (s? t:f=→"Left Max":dbl)
      }
    }
  }
  n101 = register-events(refnum<vi> refnum, w19) -> (reference out=w39:refnum<event-registration>, error out=w38:errorcluster)  [unwired: 2 in]
  n102 = call "Initialize Camera and CheckList.vi"("ListBox in"=w27) -> ()  [unwired: 11 in]
  n103 = call "Handle Camera Configuration.vi"("CameraNameRef"=w7, "Camera File Name"="Right", "ClusterRef"=w8) -> ()  [unwired: 9 in]
  n104 = while {
    tunnel: w31 -> [w230]
    tunnel: w25 -> [w228]
    tunnel: [w226] -> _
    tunnel: u32 1000 ("milliseconds to wait") -> [w225]
    tunnel: w19 -> [w219]
    i -> [w226]
    stop <- FALSE stop-if-true
    n105 = local read "Rec Mode"() -> (w221:enum32{"Stop", "Record", "Playback"})
    n106 = Wait on Notification(notifier=w228, timeout in ms (-1)=w225) -> (notification=w227:string, timed out?=w223:bool)  [unwired: 2 in, 2 out]
    n107 = Equal?(x=w221, y=u16 2 ("Rec Mode")) -> (x = y?=w222:bool)
    n108 = Compound Arithmetic op=OR(invert w223, w222) -> (w224:bool)
    n109 = case shown="True" w224 {
      tunnel: w230 -> [_ w233]
      tunnel: w227 -> [_ w232]
      tunnel: w219 -> [_ w231]
      frame False {
      }
      frame True {
        n110 = call <vilib>:"Bind Controls to SmartDashboard.vi"("RPC ref"=w231, "Bound Control Refs"=w233, "Server IP Address"=w232) -> ()  [unwired: 9 in]
      }
    }
  }
  n111 = vi-ref "Playback Controls.vi"() -> (w40:refnum<vi>)
  n112 = Bundle("Command Params"=w4, "Test Mode Array"=w2) -> (w3:T41)  [unwired: 1 in]
  n113 = property class="VI"() -> ("Panel"=w42:refnum<vi>)  [unwired: 2 in, 2 out]
  n114 = property class="Pnl"(reference=w42) -> ("Panes[]"=w43:refnum<vi>[])  [unwired: 1 in, 2 out]
  n115 = while {
    tunnel: w10 -> [w244]
    tunnel: w9 -> [_]
    tunnel: [w238] -> _
    i -> [w238]
    stop <- FALSE stop-if-true
    n116 = local read "Rec Mode"() -> (w242:enum32{"Stop", "Record", "Playback"})
    n117 = local read "Robot IP"() -> (w243:string)
    n118 = call <vilib>:"WPI_CameraRead MJPG for Dashboard.vi"("Camera Settings"="Camera Settings Right", "Rec Mode"=w242, "NT Connection"=w243, "Capture Info"="Camera Name Right", "Refnum in"=w244) -> ("Active"=w237:bool, "Refnum out"=w240:T5, "FPS"=w235:dbl, "Bandwidth (Mbps)"=w236:dbl)  [unwired: 3 in]
    n119 = case shown="False" w237 {
      tunnel: w240 -> [w246 w248]
      tunnel: w236 -> [_ _]
      tunnel: w235 -> [_ _]
      tunnel: [w246 w248] -> w234
      frame False {
        n120 = Wait Until Next ms Multiple(millisecond multiple=u32 500) -> ()  [unwired: 1 out]
      }
      frame True {
      }
    }
    "Camera Image Right" <- w234
  }
  n121 = while {
    tunnel: w50 -> [w258]
    tunnel: w49 -> [_]
    tunnel: [w259] -> _
    i -> [w259]
    stop <- FALSE stop-if-true
    # "Optionally read the DB image,\nlog, or retrieve images from a\nlogged match"
    n122 = local read "Rec Mode"() -> (w254:enum32{"Stop", "Record", "Playback"})
    n123 = local read "Robot IP"() -> (w253:string)
    n124 = call <vilib>:"WPI_CameraRead MJPG for Dashboard.vi"("Camera Settings"="Camera Settings", "Rec Mode"=w254, "NT Connection"=w253, "Capture Info"="Camera Name", "Refnum in"=w258) -> ("Active"=w256:bool, "Refnum out"=w257:T5, "FPS"=w255:dbl, "Bandwidth (Mbps)"=w252:dbl)  [unwired: 3 in]
    n125 = case shown="True" w256 {
      tunnel: w257 -> [w261 w272]
      tunnel: w252 -> [_ w269]
      tunnel: w255 -> [_ w270]
      tunnel: [w261 w266] -> w249
      frame False {
        w263 = u32 1985280 ("Color Box")
        # "Sleep for 500ms"
        n126 = Bundle("Color Box"=w263, "Color Box"=w263) -> (w264:cluster{"Color Box":u32, "Color Box":u32})  [unwired: 1 out]
        n127 = Build Array(w264) -> (w262:cluster{"Color Box":u32, "Color Box":u32}[])
        n128 = property on="Mbps LED" class="Bool (strict)"("Colors [4]"=w262) -> ()  [unwired: 2 in, 2 out]
        n129 = Wait Until Next ms Multiple(millisecond multiple=u32 500) -> ()  [unwired: 1 out]
      }
      frame True {
        # "Here is where you would annotate,\npossibly process, and display the image"
        # "Update Mbps LED"
        n130 = case shown="Default" w269 {
          tunnel: [u32 6618880 ("Color Box") u32 16776722 ("Color Box") u32 16716800 ("Color Box")] -> w273
          frame Default {
          }
          frame 4, 5 {
          }
          frame 6.. {
          }
        }
        n131 = call "IMAQ Clear Overlay"("Image"=w272) -> ("error out"=w275:errorcluster, "Image Out"=w266:T5)  [unwired: 2 in, 7 out]
        n132 = Bundle(FALSE, "Bandwidth (Mbps)"=w269, "FPS"=w270) -> (→"Camera Info":cluster{bool, "Bandwidth (Mbps)":dbl, "FPS":dbl})  [unwired: 1 in]
        n133 = Bundle("Color Box"=w273, "Color Box"=w273) -> (w274:cluster{"Color Box":u32, "Color Box":u32})  [unwired: 1 out]
        n134 = Unbundle By Name(w275) -> ("status"=w276:bool)
        n135 = Build Array(w274) -> (w271:cluster{"Color Box":u32, "Color Box":u32}[])
        n136 = property on="Image Message" class="Str"("Visible"=w276) -> ()  [unwired: 2 in, 2 out]
        n137 = property on="Mbps LED" class="Bool (strict)"("Colors [4]"=w271) -> ()  [unwired: 2 in, 2 out]
      }
    }
    "Camera Image" <- w249
  }
  n138 = Index Array(array=w43) -> (element=w41:refnum<vi>)  [unwired: 1 in]
  n139 = control-ref of="Test Tree"() -> (w44:refnum<vi>)
  n140 = while {
    tunnel: w41 -> [w281]
    i -> [w284]
    stop <- FALSE stop-if-true
    n141 = Wait (ms)(milliseconds to wait=u32 100) -> ()  [unwired: 1 out]
    n142 = case shown="\"Playback\"" "Rec Mode" {
      tunnel: w284 -> [_ _ w299]
      tunnel: [u32 2829099 ("Base Color") u32 11141120 ("Target Color") w288] -> w280
      frame "Stop", Default {
        # "Reset the color, extra updates don't cost much"
      }
      frame "Record" {
      }
      frame "Playback" {
        # "Playback"
        n143 = Quotient & Remainder(x=w299, y=u32 50 ("milliseconds to wait")) -> (x-y*floor(x/y)=w295:u32)  [unwired: 1 out]
        n144 = Divide(x=w295, y=u32 50 ("milliseconds to wait")) -> (x/y=w292:dbl)
        n145 = Multiply(x=6.283185307179586, y=w292) -> (x*y=w297:dbl)
        n146 = Sine(x=w297) -> (sin(x)=w296:dbl)
        n147 = Absolute Value(x=w296) -> (abs(x)=w289:dbl)
        n148 = call "Interpolate RGB Color.vi"("Proportion"=w289, "Target Color"=u32 30976, "Base Color"=u32 2829099) -> ("Result Color"=w288:u32)  [unwired: 8 in]
      }
    }
    n149 = property class="Pane"(reference=w281, "PaneColor"=w280) -> ()  [unwired: 1 in, 2 out]
  }
  n150 = while {
    tunnel: [w309] -> _
    tunnel: w44 -> [w308]
    tunnel: w40 -> [w307]
    tunnel: w39 -> [w306]
    tunnel: w38 -> [_]
    tunnel: w34 -> [w305]
    tunnel: w19 -> [w304]
    tunnel: w18 -> [w303]
    shift-right: [w302] -> _
    shift-left: w3 -> [w301]
    tunnel: w15 -> [w300]
    i -> [w309]
    stop <- FALSE stop-if-true
    n151 = event shown="[0] Timeout" {
      selector: w306 -> [_ _ _ _ _ _ _ _ _ _ _ _ _ _ _ _ _ _ _ _ _]
      dyn-events: [_ _ _ _ _ _ _ _ _ _ _ _ _ _ _ _ w567 _ _ _ _] -> _
      timeout: u32 60 ("milliseconds to wait") -> [_ _ _ _ _ _ _ _ _ _ _ _ _ _ _ _ _ _ _ _ _]
      tunnel: w308 -> [w319 _ _ _ _ _ _ _ _ _ _ _ _ _ _ _ _ _ _ _ _]
      tunnel: "Test Tree" -> [_ _ _ _ _ _ _ _ _ _ _ w534 w542 w544 w548 w556 _ _ _ _ _]
      tunnel: w307 -> [_ _ _ _ _ _ _ _ _ _ _ _ _ _ _ _ w569 _ w587 _ _]
      tunnel: w305 -> [_ _ _ _ _ _ _ _ _ _ _ _ _ _ _ _ w565 _ _ _ _]
      tunnel: w304 -> [_ _ _ _ _ _ _ _ _ _ _ _ _ _ _ _ w561 _ _ _ _]
      tunnel: w303 -> [w317 _ _ _ _ _ w481 _ _ _ _ _ _ _ _ _ _ _ _ _ _]
      tunnel: [w314 w358 w460 w465 w474 w478 w479 w483 w497 w509 w521 w533 w540 w543 w547 w555 w560 w582 w584 w589 w600] -> w302
      tunnel: w301 -> [w314 w358 w460 w465 w474 w478 w479 w485 w498 w509 w521 w533 w540 w543 w547 w555 w560 w582 w584 w589 w600]
      tunnel: w300 -> [w315 _ _ _ _ _ _ _ _ _ _ _ _ _ _ _ _ _ _ _ _]
      event Timeout {
        n152 = event-data() -> ()  [unwired: 1 in, 1 out]
        n153 = Unbundle By Name(w314) -> ("Test Mode Array"=w313:T9)
        n154 = case shown="\"Power\"" "Dashboard Tab" {
          tunnel: w319 -> [_ _ _ _ _ _ w335 _ _ _]
          tunnel: "/TestMode/Automatic/" ("Name Pattern") -> [_ _ _ _ _ _ w334 _ _ _]
          tunnel: w313 -> [_ _ _ _ _ _ w327 _ w352 _]
          tunnel: w317 -> [_ _ _ _ _ _ _ _ w346 _]
          tunnel: w315 -> [_ _ _ _ _ w321 _ _ _ _]
          frame "General" {
          }
          frame "Profile" {
          }
          frame "Camera" {
          }
          frame "Drive" {
          }
          frame "Power" {
          }
          frame "Basic" {
            n155 = call <vilib>:"WPI_DashboardUpdateNames.vi"("Controls on Tab"=w321) -> ()  [unwired: 11 in]
          }
          frame "Test" {
            w333 = -2 ("Active Item:Row Number")
            n156 = local read "Mode"() -> (w322:T4)
            n157 = Index Array(array=w327, index=w322) -> (element=w328:T44)
            n158 = Unbundle(w328) -> ("Operation"=w329:enum16{"Update", "Clear"}, "Color Box"=w330:u32)
            n159 = call <vilib>:"NT Read String.vi"("Name"="/TestMode/TestName") -> ("String"=w325:string)  [unwired: 9 in, 1 out]
            n160 = call <vilib>:"NT Read and Format Entries as Tree.vi"("Operation"=w329, "Name Pattern"=w334, "Tree Refnum"=w335) -> ()  [unwired: 7 in, 2 out]
            n161 = case shown="\"\"" w325 {
              tunnel: "/TestMode/TestProgress" ("Name") -> [w337 _]
              tunnel: "/TestMode/TestProgressText" ("Name") -> [w336 _]
              frame Default {
                n162 = call <vilib>:"NT Read Number.vi"("Name"=w337) -> ("Numeric"=w338:dbl)  [unwired: 9 in, 1 out]
                n163 = call <vilib>:"NT Read String.vi"("Name"=w336) -> ("String"=w339:string)  [unwired: 9 in, 1 out]
                n164 = Bundle("Numeric"=w338, "String"=w339) -> (→"Progress":cluster{"Numeric":dbl, "String":string})  [unwired: 1 in]
              }
              frame "" {
                n165 = property on="Progress" class="Clust (strict)"("Visible"=FALSE) -> ()  [unwired: 2 in, 2 out]
                n166 = local write "Test Name"(u16 0) -> ()
              }
            }
            n167 = property on="Test Tree" class="Tree (strict)"("Active Item Row Number"=w333, "ActiveColNum"=w333, "CellBG"=w330, "Active Item Row Number"=-1 ("Active Item:Row Number"), "CellBG"=u32 5789784 ("Color Box")) -> ()  [unwired: 2 in, 2 out]
          }
          frame "Variables" {
            n168 = control-ref of="Tree"() -> (w343:refnum<vi>)
            n169 = call <vilib>:"NT Read and Format Entries as Tree.vi"("Tree Refnum"=w343) -> ()  [unwired: 9 in, 2 out]
          }
          frame "Commands" {
            w353 = u32 5789784 ("Color Box")
            w354 = T17 {"Row"=-1, "Column"=-2} ("Active Cell:Active Cell")
            w356 = T17 {"Row"=-2, "Column"=-2} ("Active Cell:Active Cell")
            n170 = local read "Mode"() -> (w344:T4)
            n171 = Index Array(array=u32[] [15790320, 15790320, 15790320, 15790320, 16777215, 16777215, 15790320, 15790320, 15790320], index=w344) -> (element=w355:u32)
            n172 = Index Array(array=w352, index=w344) -> (element=w351:T44)
            n173 = Unbundle(w351) -> ("Operation"=w350:enum16{"Update", "Clear"})  [unwired: 1 out]
            n174 = local read "Command Selection"() -> (w349:i32)
            n175 = property on="Command Selection" class="MCListbox (strict)"("ActiveCell"=w356, "CellBG"=w355, "ActiveCell"=w354, "CellBG"=w353) -> ()  [unwired: 2 in, 2 out]
            n176 = call <vilib>:"WPI_DashboardUpdate RPC Info.vi"("Operation"=w350) -> ("update"=w348:bool, "commands"=w347:string[][])  [unwired: 9 in]
            n177 = property on="Command Selection" class="MCListbox (strict)"("ItemNames"=w347) -> ()  [unwired: 2 in, 2 out]
            n178 = property on="Command Params" class="Tbl (strict)"("Active Cell"=w356, "Cell BG Color"=w355, "Active Cell"=w354, "Cell BG Color"=w353) -> ()  [unwired: 2 in, 2 out]
            n179 = call <vilib>:"WPI_DashboardUpdate Command Params.vi"("Update"=w348, "NewVal"=w349, "Commands"=w347, "Param Tbl"=w346) -> ()  [unwired: 7 in, 1 out]
          }
          frame "Checklist" {
          }
        }
        n180 = call <vilib>:"Connextion Info.vi"() -> ("Connected"=→"NT Connection":bool)  [unwired: 10 in, 1 out]
      }
      event "Test Tree": Value Change {
        # "Show appropriate\ncontrols"
        n181 = event-data() -> ("CtlRef"=w361:refnum<vi>, "NewVal"=w359:string)  [unwired: 1 in]
        n182 = call <vilib>:"WPI_UtilitiesGetTreeIOName.vi"("NewVal"=w359, "TreeControl in"=w361) -> ("I/O Name"=w362:string)  [unwired: 9 in]
        n183 = case shown="\"Camera\"" w362 {
          selector: w362 -> [_ w369 _ w391 w400 _]
          tunnel: w359 -> [_ _ w388 w390 _ w407]
          tunnel: cluster{string[]}[] [{["640x480", "320x240", "160x120"]}, {["Auto", "Fixed indoor", "Fixed outdoor 1", "Fixed outdoor 2", "Fixed fluorescent 1", "Fixed fluorescent 2", "Hold current"]}, {["Auto", "Flicker-free 50 Hz", "Flicker-free 60 Hz", "Hold current"]}, {["None", "Prioritize frame rate", "Prioritize image quality"]}, {["Monochrome", "Color"]}] -> [_ _ _ _ _ w406]
          frame Default {
            w364 = FALSE ("Visible")
            w363 = FALSE ("Visible")
            n184 = property on="Motor" class="Clust (strict)"("Visible"=w363) -> ()  [unwired: 2 in, 2 out]
            n185 = property on="Test Ring" class="Ring (strict)"("Visible"=w363) -> ()  [unwired: 2 in, 2 out]
            n186 = property on="Rev/Fwd" class="Clust (strict)"("Visible"=w364) -> ()  [unwired: 2 in, 2 out]
            n187 = property on="On/Off" class="Bool (strict)"("Visible"=w364) -> ()  [unwired: 2 in, 2 out]
            n188 = property on="Test Slider" class="Slide (strict)"("Visible"=w364) -> ()  [unwired: 2 in, 2 out]
          }
          frame "Analog Out", "Motor", "PWM" {
            w370 = FALSE ("Visible")
            n189 = case shown="\"Analog Out\"" w369 {
              tunnel: [1.0 ("Value") -1.0 ("Value") 0.0 ("Value")] -> w368
              tunnel: [255.0 ("Value") 1.0 ("Value") 5.0 ("Value")] -> w367
              tunnel: [128.0 ("Value") 0.0 ("Value") 0.0 ("Value")] -> w366
              tunnel: [64.0 ("Value") 0.5 ("Value") 1.0 ("Value")] -> w365
              frame "PWM" {
              }
              frame "Motor", Default {
              }
              frame "Analog Out" {
              }
            }
            n190 = property on="Motor" class="Clust (strict)"("Visible"=TRUE) -> ()  [unwired: 2 in, 2 out]
            n191 = property on="Value" class="Slide (strict)"("Value"=w366, "Scale.Minimum"=w368, "Scale.Maximum"=w367, "Scale.Increment"=w365) -> ()  [unwired: 2 in, 2 out]
            n192 = property on="On/Off" class="Bool (strict)"("Visible"=w370) -> ()  [unwired: 2 in, 2 out]
            n193 = property on="Test Slider" class="Slide (strict)"("Visible"=w370) -> ()  [unwired: 2 in, 2 out]
            n194 = property on="Test Ring" class="Ring (strict)"("Visible"=w370) -> ()  [unwired: 2 in, 2 out]
            n195 = property on="Rev/Fwd" class="Clust (strict)"("Visible"=w370) -> ()  [unwired: 2 in, 2 out]
          }
          frame "Servo" {
            w386 = FALSE ("Visible")
            n196 = call <vilib>:"NT Read Number.vi"("Name"=w388) -> ("Numeric"=w387:dbl)  [unwired: 9 in, 1 out]
            n197 = property on="Test Slider" class="Slide (strict)"("Visible"=TRUE, "Scale.Maximum"=170.0 ("Scale.Range:Maximum")) -> ()  [unwired: 2 in, 2 out]
            n198 = local write "Test Slider"(w387) -> ()
            n199 = property on="Motor" class="Clust (strict)"("Visible"=w386) -> ()  [unwired: 2 in, 2 out]
            n200 = property on="Rev/Fwd" class="Clust (strict)"("Visible"=w386) -> ()  [unwired: 2 in, 2 out]
            n201 = property on="On/Off" class="Bool (strict)"("Visible"=w386) -> ()  [unwired: 2 in, 2 out]
            n202 = property on="Test Ring" class="Ring (strict)"("Visible"=w386) -> ()  [unwired: 2 in, 2 out]
          }
          frame "Relay", "Solenoid" {
            w389 = FALSE ("Visible")
            n203 = property on="Motor" class="Clust (strict)"("Visible"=w389) -> ()  [unwired: 2 in, 2 out]
            n204 = property on="Test Slider" class="Slide (strict)"("Visible"=w389) -> ()  [unwired: 2 in, 2 out]
            n205 = Search and Replace String(input string=w390, search string="/Value  **", replace string="/Direction") -> (result string=w396:string)  [unwired: 5 in, 3 out]
            n206 = property on="Test Ring" class="Ring (strict)"("Visible"=w389) -> ()  [unwired: 2 in, 2 out]
            n207 = call <vilib>:"NT Read String.vi"("Name"=w396) -> ("String"=w394:string)  [unwired: 9 in, 1 out]
            n208 = Equal?(x="Both directions", y=w394) -> (x = y?=w392:bool)
            n209 = Not(x=w392) -> (.not. x?=w393:bool)
            n210 = property on="Rev/Fwd" class="Clust (strict)"("Visible"=w392) -> ()  [unwired: 2 in, 2 out]
            n211 = property on="On/Off" class="Bool (strict)"("Visible"=w393, "Caption.Text"=w391) -> ()  [unwired: 2 in, 2 out]
          }
          frame "Compressor", "Digital Out" {
            w399 = FALSE ("Visible")
            # "Get direction and finish"
            n212 = property on="Motor" class="Clust (strict)"("Visible"=w399) -> ()  [unwired: 2 in, 2 out]
            n213 = property on="Test Slider" class="Slide (strict)"("Visible"=w399) -> ()  [unwired: 2 in, 2 out]
            n214 = property on="Test Ring" class="Ring (strict)"("Visible"=w399) -> ()  [unwired: 2 in, 2 out]
            n215 = property on="On/Off" class="Bool (strict)"("Visible"=TRUE, "Caption.Text"=w400) -> ()  [unwired: 2 in, 2 out]
            n216 = property on="Rev/Fwd" class="Clust (strict)"("Visible"=FALSE) -> ()  [unwired: 2 in, 2 out]
          }
          frame "Camera" {
            n217 = call <vilib>:"Get Last Path Segment.vi"("String in"=w407) -> ("String out"=w408:string)  [unwired: 10 in]
            n218 = property on="On/Off" class="Bool (strict)"("Visible"=FALSE) -> ()  [unwired: 2 in, 2 out]
            n219 = property on="Motor" class="Clust (strict)"("Visible"=FALSE) -> ()  [unwired: 2 in, 2 out]
            n220 = property on="Rev/Fwd" class="Clust (strict)"("Visible"=FALSE) -> ()  [unwired: 2 in, 2 out]
            n221 = case shown="\"White Balance  **\"" w408 {
              tunnel: w407 -> [w414 w423 w432 w441 w450 _ w456]
              tunnel: w406 -> [w412 w420 w429 w438 w447 _ _]
              frame "Size  **" {
                n222 = Index Array(array=w412) -> (element=w411:cluster{string[]})  [unwired: 1 in]
                n223 = call <vilib>:"NT Read String.vi"("Name"=w414) -> ("String"=w413:string)  [unwired: 9 in, 1 out]
                n224 = Unbundle(w411) -> (w409:string[])
                n225 = Match First String(2:w409, 3:w413) -> (0:w410:i32)  [unwired: 1 out]
                n226 = property on="Test Ring" class="Ring (strict)"("Value"=w410, "Strings []"=w409) -> ()  [unwired: 2 in, 2 out]
                n227 = property on="Test Ring" class="Ring (strict)"("Visible"=TRUE) -> ()  [unwired: 2 in, 2 out]
                n228 = property on="Test Slider" class="Slide (strict)"("Visible"=FALSE) -> ()  [unwired: 2 in, 2 out]
              }
              frame "White Balance  **" {
                n229 = Index Array(array=w420, index=1) -> (element=w421:cluster{string[]})
                n230 = call <vilib>:"NT Read String.vi"("Name"=w423) -> ("String"=w422:string)  [unwired: 9 in, 1 out]
                n231 = Unbundle(w421) -> (w418:string[])
                n232 = Match First String(2:w418, 3:w422) -> (0:w417:i32)  [unwired: 1 out]
                n233 = property on="Test Ring" class="Ring (strict)"("Value"=w417, "Strings []"=w418) -> ()  [unwired: 2 in, 2 out]
                n234 = property on="Test Ring" class="Ring (strict)"("Visible"=TRUE) -> ()  [unwired: 2 in, 2 out]
                n235 = property on="Test Slider" class="Slide (strict)"("Visible"=FALSE) -> ()  [unwired: 2 in, 2 out]
              }
              frame "Exposure  **" {
                n236 = Index Array(array=w429, index=2) -> (element=w430:cluster{string[]})
                n237 = call <vilib>:"NT Read String.vi"("Name"=w432) -> ("String"=w431:string)  [unwired: 9 in, 1 out]
                n238 = Unbundle(w430) -> (w426:string[])
                n239 = Match First String(2:w426, 3:w431) -> (0:w427:i32)  [unwired: 1 out]
                n240 = property on="Test Ring" class="Ring (strict)"("Value"=w427, "Strings []"=w426) -> ()  [unwired: 2 in, 2 out]
                n241 = property on="Test Ring" class="Ring (strict)"("Visible"=TRUE) -> ()  [unwired: 2 in, 2 out]
                n242 = property on="Test Slider" class="Slide (strict)"("Visible"=FALSE) -> ()  [unwired: 2 in, 2 out]
              }
              frame "Exposure Priority  **" {
                n243 = Index Array(array=w438, index=3) -> (element=w439:cluster{string[]})
                n244 = call <vilib>:"NT Read String.vi"("Name"=w441) -> ("String"=w440:string)  [unwired: 9 in, 1 out]
                n245 = Unbundle(w439) -> (w435:string[])
                n246 = Match First String(2:w435, 3:w440) -> (0:w436:i32)  [unwired: 1 out]
                n247 = property on="Test Ring" class="Ring (strict)"("Value"=w436, "Strings []"=w435) -> ()  [unwired: 2 in, 2 out]
                n248 = property on="Test Ring" class="Ring (strict)"("Visible"=TRUE) -> ()  [unwired: 2 in, 2 out]
                n249 = property on="Test Slider" class="Slide (strict)"("Visible"=FALSE) -> ()  [unwired: 2 in, 2 out]
              }
              frame "Color Enable  **" {
                n250 = Index Array(array=w447, index=4) -> (element=w448:cluster{string[]})
                n251 = call <vilib>:"NT Read String.vi"("Name"=w450) -> ("String"=w449:string)  [unwired: 9 in, 1 out]
                n252 = Unbundle(w448) -> (w444:string[])
                n253 = Match First String(2:w444, 3:w449) -> (0:w445:i32)  [unwired: 1 out]
                n254 = property on="Test Ring" class="Ring (strict)"("Value"=w445, "Strings []"=w444) -> ()  [unwired: 2 in, 2 out]
                n255 = property on="Test Ring" class="Ring (strict)"("Visible"=TRUE) -> ()  [unwired: 2 in, 2 out]
                n256 = property on="Test Slider" class="Slide (strict)"("Visible"=FALSE) -> ()  [unwired: 2 in, 2 out]
              }
              frame Default {
                n257 = property on="Test Ring" class="Ring (strict)"("Visible"=FALSE) -> ()  [unwired: 2 in, 2 out]
                n258 = property on="Test Slider" class="Slide (strict)"("Visible"=FALSE) -> ()  [unwired: 2 in, 2 out]
              }
              frame "Brightness  **", "Color Level  **", "Compression  **", "FPS  **", "Sharpness  **" {
                n259 = call <vilib>:"NT Read Number.vi"("Name"=w456) -> ("Numeric"=w455:dbl)  [unwired: 9 in, 1 out]
                n260 = local write "Test Slider"(w455) -> ()
                n261 = property on="Test Slider" class="Slide (strict)"("Visible"=TRUE, "Scale.Maximum"=100.0 ("Scale.Range:Maximum")) -> ()  [unwired: 2 in, 2 out]
                n262 = property on="Test Ring" class="Ring (strict)"("Visible"=FALSE) -> ()  [unwired: 2 in, 2 out]
              }
            }
          }
        }
        n263 = property on="Progress" class="Clust (strict)"("Visible"=FALSE) -> ()  [unwired: 2 in, 2 out]
      }
      event "Test Name": Mouse Enter {
        # "Populate the ring with the list of tests"
        n264 = event-data() -> ()  [unwired: 1 in, 1 out]
        n265 = call <vilib>:"NT Read String Array.vi"("Name"="/TestMode/TestList") -> ("String Array"=w464:string[])  [unwired: 9 in, 1 out]
        n266 = Build Array (concatenate)("Select the test to run...", w464) -> (w463:string[])
        n267 = property on="Test Name" class="Ring (strict)"("Strings []"=w463) -> ()  [unwired: 2 in, 2 out]
      }
      event "Test Name": Value Change {
        w466 = FALSE ("Visible")
        # "Tell the robot the test name to run"
        n268 = event-data() -> ("NewVal"=w470:u16)  [unwired: 1 in]
        n269 = property on="Test Name" class="Ring (strict)"() -> ("Strings []"=w471:string[])  [unwired: 2 in, 2 out]
        n270 = local write "Progress"(T8 {"Test Progress"=0, "Test Progress Text"=""} ("Progress")) -> ()
        n271 = Index Array(array=w471, index=w470) -> (element=w469:string)
        n272 = call <vilib>:"NT Write String.vi"("String"=w469, "Name"="/TestMode/TestName") -> ()  [unwired: 9 in, 1 out]
        n273 = property on="Progress" class="Clust (strict)"("Visible"=TRUE) -> ()  [unwired: 2 in, 2 out]
        n274 = property on="Motor" class="Clust (strict)"("Visible"=w466) -> ()  [unwired: 2 in, 2 out]
        n275 = property on="Test Slider" class="Slide (strict)"("Visible"=w466) -> ()  [unwired: 2 in, 2 out]
        n276 = property on="On/Off" class="Bool (strict)"("Visible"=w466) -> ()  [unwired: 2 in, 2 out]
        n277 = property on="Rev/Fwd" class="Clust (strict)"("Visible"=w466) -> ()  [unwired: 2 in, 2 out]
        n278 = property on="Test Ring" class="Ring (strict)"("Visible"=w466) -> ()  [unwired: 2 in, 2 out]
      }
      event "Select Auto": Mouse Enter {
        # "Populate the combo box with the list of autonomous options"
        n279 = event-data() -> ()  [unwired: 1 in, 1 out]
        n280 = call <vilib>:"NT Read String Array.vi"("Name"="Auto List") -> ("String Array"=w473:string[])  [unwired: 9 in, 1 out]
        n281 = property on="Select Auto" class="CmbBox"("Strings[]"=w473) -> ()  [unwired: 2 in, 2 out]
      }
      event "Select Auto": Value Change {
        # "User modified the Auto Selection. Write to NT variable so robot knows."
        n282 = event-data() -> ("NewVal"=w476:string)  [unwired: 1 in]
        n283 = call <vilib>:"NT Write String.vi"("String"=w476, "Name"="Auto Selector") -> ()  [unwired: 9 in, 1 out]
      }
      event "Command Selection": Value Change {
        # "Get the params and show in table"
        n284 = event-data() -> ("NewVal"=w482:i32)  [unwired: 1 in]
        n285 = property on="Command Selection" class="MCListbox (strict)"() -> ("ItemNames"=w480:string[][])  [unwired: 2 in, 2 out]
        n286 = call <vilib>:"WPI_DashboardUpdate Command Params.vi"("NewVal"=w482, "Commands"=w480, "Param Tbl"=w481) -> ()  [unwired: 8 in, 1 out]
      }
      event "Execute Command": Value Change {
        # "Started one, Unique ID holds\nresponse"
        n287 = event-data() -> ()  [unwired: 1 in, 1 out]
        n288 = property on="Command Selection" class="MCListbox (strict)"() -> ("ItemNames"=w495:string[][])  [unwired: 2 in, 2 out]
        n289 = Index Array(array=w495, index (row)="Command Selection", index (col)=0) -> (element=w493:string)
        n290 = call <vilib>:"Invoke Commands.vi"("Command Params"="Command Params", "Function Name"=w493) -> ("Params"=w490:u8, "Started"=w489:bool)  [unwired: 7 in, 1 out]
        n291 = Array Subset(array="Command Params", length (row)=w490) -> (w484:string[][])  [unwired: 3 in]
        n292 = Bundle By Name(cluster=w485, "Command Params"=w484) -> (w483:T41)
        n293 = Select(t="Executing" ("Cmd Status"), s=w489, f="" ("Cmd Status")) -> (s? t:f=→"Cmd Status":string)
      }
      event "Command Selection": Double Click {
        n294 = event-data() -> ("Row"=w505:i32)  [unwired: 1 in]
        n295 = property on="Command Selection" class="MCListbox (strict)"() -> ("ItemNames"=w508:string[][])  [unwired: 2 in, 2 out]
        n296 = local read "Command Params"() -> (w504:string[][])
        n297 = Index Array(array=w508, index (row)=w505, index (col)=0) -> (element=w506:string)
        n298 = call <vilib>:"Invoke Commands.vi"("Command Params"=w504, "Function Name"=w506) -> ("Params"=w503:u8, "Started"=w499:bool)  [unwired: 7 in, 1 out]
        n299 = Array Subset(array=w504, length (row)=w503) -> (w496:string[][])  [unwired: 3 in]
        n300 = Bundle By Name(cluster=w498, "Command Params"=w496) -> (w497:T41)
        n301 = Select(t="Executing" ("Cmd Status"), s=w499, f="" ("Cmd Status")) -> (s? t:f=w500:string)
        n302 = local write "Cmd Status"(w500) -> ()
      }
      event "CheckList": Double Click {
        # "Shift clears all"
        # "Update symbols on the listbox"
        n303 = event-data() -> ("PlatMods.Shift"=w510:bool, "Row"=w512:i32)  [unwired: 1 in]
        n304 = case shown="True" w510 {
          tunnel: w512 -> [w516 _]
          tunnel: 1 -> [w515 _]
          frame False {
            n305 = property on="CheckList" class="LstBox (strict)"() -> ("Item Symbols"=w514:i32[])  [unwired: 2 in, 2 out]
            n306 = Replace Array Subset(array=w514, new element=w515, index=w516) -> (w513:i32[])
            n307 = property on="CheckList" class="LstBox (strict)"("Item Symbols"=w513) -> ()  [unwired: 2 in, 2 out]
          }
          frame True {
            w517 = 0 ("Top Row")
            n308 = property on="CheckList" class="LstBox (strict)"() -> ("Number of Rows"=w519:u32)  [unwired: 2 in, 2 out]
            n309 = Initialize Array(0, w519) -> (w518:i32[])
            n310 = property on="CheckList" class="LstBox (strict)"("Top Row"=w517, "Value"=w517, "Item Symbols"=w518) -> ()  [unwired: 2 in, 2 out]
          }
        }
      }
      event "CheckList": Key Down {
        # "Update symbols on the listbox\nLeft and right keys check and uncheck"
        n311 = event-data() -> ("VKey"=w523:T42)  [unwired: 1 in]
        n312 = case shown="Default" w523 {
          selector: w523 -> [w528 _]
          tunnel: eventvkey."Left" ("VKey") -> [w526 _]
          frame "Left", "Right" {
            n313 = Equal?(x=w526, y=w528) -> (x = y?=w527:bool)
            n314 = Select(t=0, s=w527, f=1) -> (s? t:f=w529:i32)
            n315 = property on="CheckList" class="LstBox (strict)"() -> ("Item Symbols"=w532:i32[])  [unwired: 2 in, 2 out]
            n316 = Replace Array Subset(array=w532, new element=w529, index="CheckList") -> (w531:i32[])
            n317 = property on="CheckList" class="LstBox (strict)"("Item Symbols"=w531) -> ()  [unwired: 2 in, 2 out]
          }
          frame Default {
          }
        }
      }
      event "Motor.Enable": Value Change {
        # "When the test mode otor enable helper is set, update that\ntree row item's value"
        n318 = event-data() -> ("NewVal"=w538:bool)  [unwired: 1 in]
        n319 = Unbundle("Motor") -> ("Value"=w537:dbl)  [unwired: 1 out]
        n320 = Select(t=w537, s=w538, f=0.0) -> (s? t:f=w535:dbl)
        n321 = call <vilib>:"NT Write Number.vi"("Numeric"=w535, "Name"=w534) -> ()  [unwired: 9 in, 1 out]
      }
      event "Test Slider": Value Change {
        # "When the test mode slider helper is set, update that\ntree row item's value"
        n322 = event-data() -> ("NewVal"=w541:dbl)  [unwired: 1 in]
        n323 = call <vilib>:"NT Write Number.vi"("Numeric"=w541, "Name"=w542) -> ()  [unwired: 9 in, 1 out]
      }
      event "On/Off": Value Change {
        # "When the test mode on/off helper value is set, update that\ntree row item's value"
        n324 = event-data() -> ("NewVal"=w546:bool)  [unwired: 1 in]
        n325 = Boolean To (0,1)(Boolean=w546) -> (0, 1=w545:i16)
        n326 = call <vilib>:"NT Write Number.vi"("Numeric"=w545, "Name"=w544) -> ()  [unwired: 9 in, 1 out]
      }
      event "Rev/Fwd": Value Change {
        # "When the test mode helper value for relays is set, update that\ntree row item's value"
        n327 = event-data() -> ("NewVal.Forward"=w554:bool, "NewVal.Reverse"=w553:bool)  [unwired: 1 in]
        n328 = Boolean To (0,1)(Boolean=w554) -> (0, 1=w550:i16)
        n329 = Boolean To (0,1)(Boolean=w553) -> (0, 1=w552:i16)
        n330 = Negate(x=w552) -> (-x=w551:i16)
        n331 = Add(x=w550, y=w551) -> (x+y=w549:i16)
        n332 = call <vilib>:"NT Write Number.vi"("Numeric"=w549, "Name"=w548) -> ()  [unwired: 9 in, 1 out]
      }
      event "Test Ring": Value Change {
        # "When a test mode helper value is selected from the ring,\nset the tree item's variable to the string value"
        n333 = event-data() -> ("NewVal"=w558:u16)  [unwired: 1 in]
        n334 = property on="Test Ring" class="Ring (strict)"() -> ("Strings []"=w559:string[])  [unwired: 2 in, 2 out]
        n335 = Index Array(array=w559, index=w558) -> (element=w557:string)
        n336 = call <vilib>:"NT Write String.vi"("String"=w557, "Name"=w556) -> ()  [unwired: 9 in, 1 out]
      }
      event "Rec Mode": Value Change {
        # "Update globals for recording mode and path to read log from.\nClear when logging and let NetworkTables set path for vision to\nuse."
        n337 = event-data() -> ("NewVal"=w570:enum32{"Stop", "Record", "Playback"})  [unwired: 1 in]
        n338 = global write "WPI_DashboardLogging Global.vi" "Logging Filename"(path "") -> ()
        n339 = global write "WPI_DashboardLogging Global.vi" "Recording"(w570) -> ()
        n340 = case shown="\"Playback\"" w570 {
          tunnel: w569 -> [_ w572 w581]
          tunnel: [_ _ w580] -> w567
          tunnel: [_ _ w579] -> _
          tunnel: w565 -> [_ _ w577]
          tunnel: cluster{i32, i32} {-250, 170} -> [_ _ w576]
          tunnel: [_ _ T43 {"Image Size"=TRUE, "Image Type"=TRUE, "Pixel Value"=TRUE, "ROI Information"=TRUE, "Zoom Factor"=FALSE} ("Image Information Shown:All Elements")] -> w563
          tunnel: [_ _ TRUE ("Zoom Factor")] -> w562
          tunnel: w561 -> [_ _ w573]
          frame Default {
          }
          frame "Stop", "Record" {
            # "Place Window too"
            n341 = invoke class="VI" method="FP.Close"(reference=w572) -> (reference out=w571:refnum<vi>)  [unwired: 2 in, 2 out]
            n342 = invoke class="VI" method="Abort VI"(reference=w571) -> ()  [unwired: 2 in, 3 out]
          }
          frame "Playback" {
            n343 = call "Open Playback Panel.vi"("Offset"=w576, "DB VI Ref"=w577, "Playback in"=w581) -> ("Playback out"=w578:refnum<vi>)  [unwired: 8 in]
            n344 = register-events(w578, w573) -> (reference out=w580:refnum<event-registration>, error out=w579:errorcluster)  [unwired: 2 in]
          }
        }
        n345 = property on="Camera Image" class="ImageControl"("Image Information Shown"=w563, "Image Information Visible"=w562) -> ()  [unwired: 2 in, 2 out]
        n346 = call <vilib>:"WPI_DashboardNT Log FieldName Cache.vi"("Operation"=enum16{"Lookup/Add", "Index", "Clear"}."Clear") -> ()  [unwired: 8 in, 3 out]
      }
      event Panel Close {
        w583 = enum32{"Stop", "Record", "Playback"}."Stop" ("Rec Mode")
        # "Playback window has been closed, abort"
        n347 = event-data() -> ()  [unwired: 1 in, 4 out]
        n348 = local write "Rec Mode"(w583) -> ()
        n349 = global write "WPI_DashboardLogging Global.vi" "Recording"(w583) -> ()
      }
      event Panel Close {
        # "Abort playback window and ourself"
        n350 = event-data() -> ()  [unwired: 1 in, 4 out]
        n351 = invoke class="VI" method="FP.Close"(reference=w587) -> (reference out=w586:refnum<vi>)  [unwired: 2 in, 2 out]
        n352 = invoke class="VI" method="Abort VI"(reference=w586) -> (error out=w585:errorcluster)  [unwired: 2 in, 2 out]
        n353 = invoke class="VI" method="Abort VI"(error in=w585) -> ()  [unwired: 2 in, 3 out]
      }
      event User Event {
        n354 = event-data() -> ("IDs"=w595:cluster{"RPC field ID":u16, "Unique ID":u16}, "String"=w594:string)  [unwired: 1 in]
        n355 = Unbundle By Name(w589) -> ("Command Params"=w588:string[][])
        n356 = Bundle("IDs"=w595, "String"=w594) -> (w593:T11)  [unwired: 1 in]
        n357 = call <vilib>:"Retrieve RPC Response.vi"("RPC Response"=w593) -> ("Output"=w591:string[][])  [unwired: 10 in]
        n358 = Build Array (concatenate)(w588, w591) -> (w590:string[][])
        n359 = local write "Command Params"(w590) -> ()
        n360 = local write "Cmd Status"("" ("Cmd Status")) -> ()
      }
      event "Tree": Double Click {
        n361 = event-data() -> ("PlatMods"=w599:T45, "Tag"=w598:string)  [unwired: 1 in]
        n362 = Unbundle(w599) -> ("Shift"=w597:bool)  [unwired: 4 out]
        n363 = Not(x=w597) -> (.not. x?=w596:bool)
        n364 = call <vilib>:"NT Update Persistence.vi"("Persistence"=w596, "Name"=w598) -> ()  [unwired: 9 in, 1 out]
      }
    }
  }
  n365 = while {
    tunnel: u16 1741 ("timeout ms (25000)") -> [w602]
    stop <- FALSE stop-if-true
    n366 = TCP Create Listener(10:w602) -> (0:w601:errorcluster, 3:w603:refnum<k5>)  [unwired: 4 in, 1 out]
    n367 = case shown="No Error" w601 {
      selector: w601 -> [w605 _]
      tunnel: w603 -> [w606 _]
      frame No Error {
        n368 = while {
          tunnel: w606 -> [w609]
          tunnel: w605 -> [w608]
          stop <- FALSE stop-if-true
          n369 = TCP Wait On Listener(8:w608, 11:w609) -> (0:w610:errorcluster, 4:w611:refnum<k5>)  [unwired: 2 in, 3 out]
          n370 = local write "TCP"(w611) -> ()
          n371 = case shown="No Error" w610 {
            frame No Error {
            }
            frame Error {
              n372 = Wait (ms)(milliseconds to wait=u32 1000) -> ()  [unwired: 1 out]
            }
          }
        }
      }
      frame Error {
        n373 = Wait (ms)(milliseconds to wait=u32 1000) -> ()  [unwired: 1 out]
      }
    }
  }
  n374 = local write "Dashboard Tab"(T2."Power" ("Dashboard Tab")) -> ()
  n375 = property on="On/Off" class="Bool (strict)"("Visible"=w26) -> ()  [unwired: 2 in, 2 out]
  n376 = property on="Motor" class="Clust (strict)"("Visible"=w26) -> ()  [unwired: 2 in, 2 out]
  n377 = property on="Progress" class="Clust (strict)"("Visible"=w26) -> ()  [unwired: 2 in, 2 out]
  n378 = property on="Test Ring" class="Ring (strict)"("Visible"=w26) -> ()  [unwired: 2 in, 2 out]
  n379 = property on="Rev/Fwd" class="Clust (strict)"("Visible"=w26) -> ()  [unwired: 2 in, 2 out]
  n380 = local write "Command Selection"(u16 0 ("milliseconds to wait")) -> ()
  n381 = local write "Command Params"(string[][] [] ("Command Params")) -> ()
  n382 = global write "WPI_DashboardLogging Global.vi" "Recording"(w35) -> ()
  n383 = local write "Rec Mode"(w35) -> ()
  n384 = call <vilib>:"NT Write String.vi"("String"="Select Auto", "Name"="Auto Selector") -> ()  [unwired: 9 in, 1 out]
